vi "Configure Sensor Acquisition.vi"(7 "I2C Channel":u8, 8 "error in (no error)":errorcluster, 9 "<SMPLRT_DIV REG> Sample Rate Divider":u8, 10 "<DLPF REG> Low Pass Filter Configuration":u8(ring) items=["LP BW: 256 Hz @Sample Rate: 8kHz", "LP BW: 188 Hz @Sample Rate: 1kHz", "LP BW:   98 Hz @Sample Rate: 1kHz", "LP BW:   42 Hz @Sample Rate: 1kHz", "LP BW:   20 Hz @Sample Rate: 1kHz", "LP BW:   10 Hz @Sample Rate: 1kHz", "LP BW:     5 Hz @Sample Rate: 1kHz"], 11 "LINX Resource In":T1) -> (0 "error out":errorcluster, 2 "Actual Sampling Frequency (Hz)":dbl, 3 "LINX Resource Out":T1)   [LabVIEW 2014, in "LMH-LINX.lvlib" / "ITG3200.lvlib"]
uses:
  <vilib>/MakerHub/LINX/Public/Sensors/Gyroscopes/ITG3200/ITG3200.lvlib
  <vilib>/MakerHub/LINX/Private/Type Defs/LINX Ref.ctl
  <vilib>/MakerHub/LINX/Private/Type Defs/Platform.ctl
  <vilib>/MakerHub/LINX/Private/Type Defs/Interface.ctl
  <vilib>/MakerHub/LINX/Private/Device/Type Defs/LINX Device Config.ctl
  <vilib>/MakerHub/LINX/Private/Device/Type Defs/TCP Config.ctl
  <vilib>/MakerHub/LINX/Private/Device/Type Defs/Channels.ctl
  <vilib>/MakerHub/LINX/Private/Local IO/LinxI2cWrite.vi
  <vilib>/MakerHub/LINX/Public/Utilities/Check Channel.vi
  <vilib>/MakerHub/LINX/Private/Utilties/Generate Error.vi
  <vilib>/MakerHub/LINX/LMH-LINX.lvlib
  <vilib>/MakerHub/LINX/Private/Device/Device.lvlib
panel:
  # "INPUTS"
  # "OUTPUTS"
  # "samples/sec"
  # "0-255"
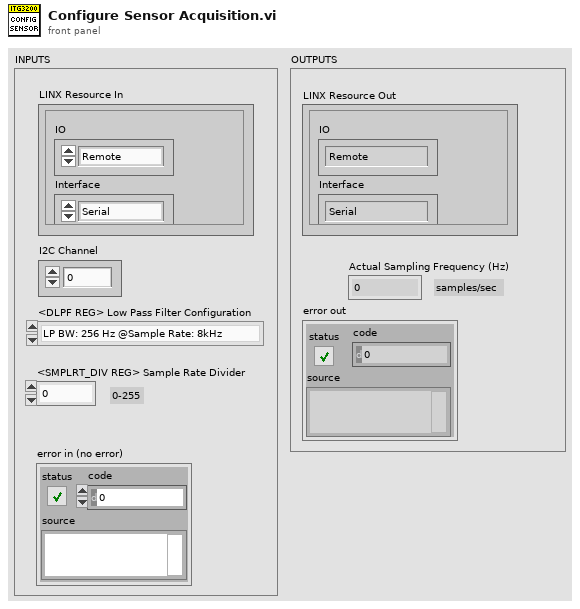
[diagram p1: front panel]
types:
  T1 = typedef "LMH-LINX.lvlib/LINX Ref.ctl" = cluster{"IO":T2, "Interface":T3, "LINX Device Config":T4}
  T2 = typedef "LMH-LINX.lvlib/Platform.ctl" = enum16{"Remote", "Local"}
  T3 = typedef "LMH-LINX.lvlib/Interface.ctl" = enum16{"Serial", "TCP"}
  T4 = typedef "LMH-LINX.lvlib/Device.lvlib/LINX Device Config.ctl" = cluster{"Interface":T3, "COM Port":refnum<visa-resource-name>, "TCP Configuration":T5, "Device Family":u8, "Device ID":u8, "Device Name":string, "TCP Ref":refnum<k5>, "Channels":T6}
  T5 = typedef "LMH-LINX.lvlib/Device.lvlib/TCP Config.ctl" = cluster{"IP Address":string, "Port":u16}
  T6 = typedef "LMH-LINX.lvlib/Channels.ctl" = cluster{"DI":u8[], "DO":u8[], "AI":u8[], "AO":u8[], "PWM":u8[], "QE":u8[], "UART":u8[], "I2C 2":u8[], "SPI":u8[], "CAN":u8[], "Servo":u8[], "AI Ref (V)":dbl, "AI Resolution (Bits)":u8, "AO Ref (V)":dbl, "AO Resolution (Bits)":u8}
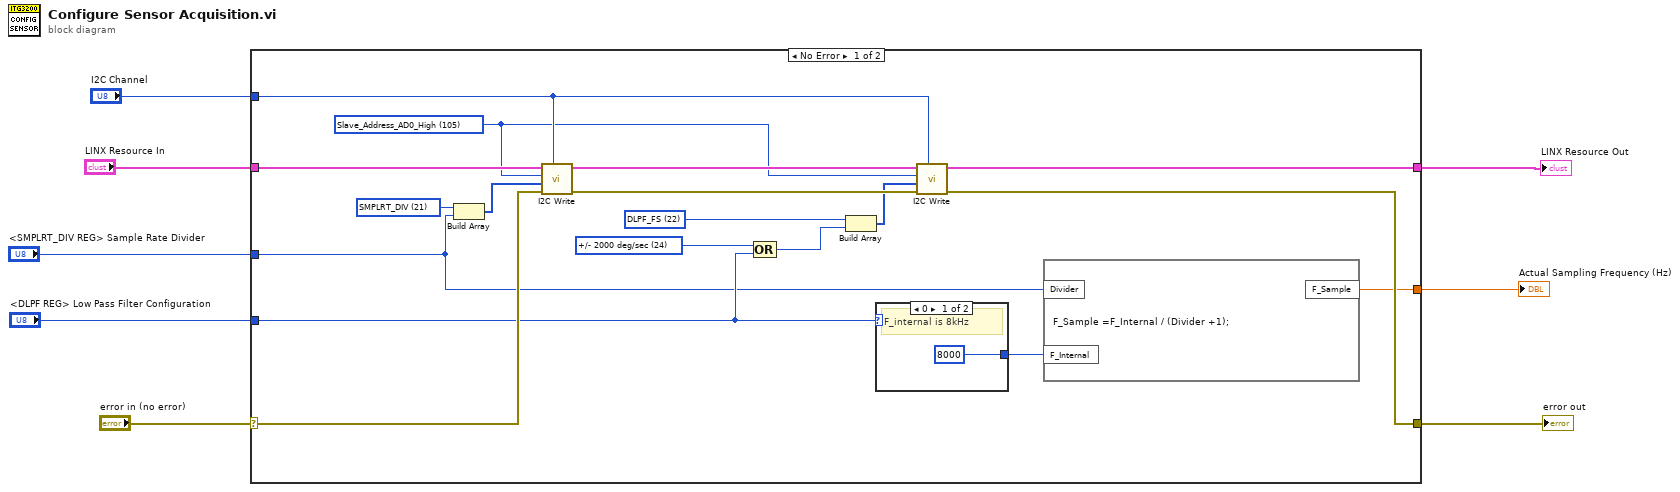
[diagram p0: block diagram]
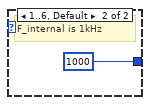
[diagram p2: hidden frame]
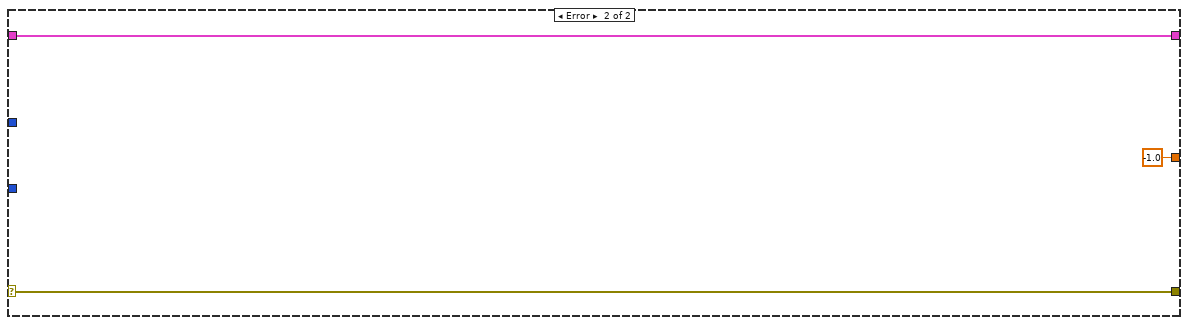
[diagram p3: hidden frame]
diagram:
  n1 = case shown="No Error" "error in (no error)" {
    selector: "error in (no error)" -> [w25 w31]
    tunnel: [w14 w31] -> w7
    tunnel: "LINX Resource In" -> [w26 w30]
    tunnel: "I2C Channel" -> [w20 _]
    tunnel: "<SMPLRT_DIV REG> Sample Rate Divider" -> [w9 _]
    tunnel: "<DLPF REG> Low Pass Filter Configuration" -> [w12 _]
    tunnel: [w13 w30] -> w2
    tunnel: [w11 -1.0 ("F_Sample")] -> w1
    frame No Error {
      w18 = u8 22 items=["WHO_AM_I"=0, "SMPLRT_DIV"=21, "DLPF_FS"=22, "INT_CFG"=23, "INT_STATUS"=26, "TEMP_OUT_H"=27, "TEMP_OUT_L"=28, "GYRO_XOUT_H"=29, "GYRO_XOUT_L"=30, "GYRO_YOUT_H"=31, "GYRO_YOUT_L"=32, "GYRO_ZOUT_H"=33, "GYRO_ZOUT_L"=34, "PWR_MGM"=62] ("Register Map")
      w16 = u8 24 items=["+/- 2000 deg/sec"=24] ("<DLPF  REG> Full Scale Select")
      w24 = u8 21 items=["WHO_AM_I"=0, "SMPLRT_DIV"=21, "DLPF_FS"=22, "INT_CFG"=23, "INT_STATUS"=26, "TEMP_OUT_H"=27, "TEMP_OUT_L"=28, "GYRO_XOUT_H"=29, "GYRO_XOUT_L"=30, "GYRO_YOUT_H"=31, "GYRO_YOUT_L"=32, "GYRO_ZOUT_H"=33, "GYRO_ZOUT_L"=34, "PWR_MGM"=62] ("Register Map")
      w19 = u8 105 items=["Slave_Address_AD0_Low"=104, "Slave_Address_AD0_High"=105] ("Slave Addresses")
      n2 = Build Array(w24, w9) -> (w23:u8[])
      n3 = call <vilib>:"I2C Write.vi"("I2C Channel"=w20, "Error In"=w25, "Data"=w23, "I2C Slave Address (0)"=w19, "LINX Resource"=w26) -> ("Error Out"=w21:errorcluster, "LINX Resource"=w22:T1)  [unwired: 5 in]
      n4 = Compound Arithmetic op=OR(w16, w12) -> (w15:u8)
      n5 = Build Array(w18, w15) -> (w17:u8[])
      n6 = case shown="0" w12 {
        tunnel: [8000 1000] -> w10
        frame 0 {
          # "F_internal is 8kHz"
        }
        frame 1..6, Default {
          # "F_internal is 1kHz"
        }
      }
      n7 = call <vilib>:"I2C Write.vi"("I2C Channel"=w20, "Error In"=w21, "Data"=w17, "I2C Slave Address (0)"=w19, "LINX Resource"=w22) -> ("Error Out"=w14:errorcluster, "LINX Resource"=w13:T1)  [unwired: 5 in]
      n8 = formula code="F_Sample =F_Internal / (Divider +1);"("Divider"=w9, "F_Internal"=w10) -> ("F_Sample"=w11:dbl)
    }
    frame Error {
    }
  }
  "error out" <- w7
  "LINX Resource Out" <- w2
  "Actual Sampling Frequency (Hz)" <- w1
